vi "Main.vi"() -> ()   [LabVIEW 2013]
uses:
  <vilib>/Utility/error.llb/DialogType.ctl
panel:
  out "setPoint V 3":string
  out "setPoint I 3":string
  out "K3 conn":bool caption="NC"
  out "setPoint V 2":string
  out "setPoint I 2":string
  out "setPoint V 1":string
  out "setPoint I 1":string
  out "message 3":string=" INSTRUCTIONS:\r\rNormal Use:  When using subVIs that incorporate the error in/error out (or error I/O) structure, place this handler where you want to inform the user of an error, typically at the end of the I/O data path, as the last action of the program.  If the error in error? is ERROR, the handler creates a message describing the error and its source.  If the type of dialog = 1 (default), the message is displayed to the user, who can only acknowedge it.  If the type = 2, the user can acknowledge the message or abort execution; aborting a program with active I/O is not recommended.  If the type = 0, no message is displayed; this is used to process the error programmatically, and the error out cluster elements are wired to individual terminals for that reason.  \r\rOther Use:\n\r\nlocal testing.  To test the error code of a subVI or function that does not have the error I/O structure, you can wire its error code and a source string to the local error code and error source inputs.  If error in error? indicates no error and error code is not equal to 0, the local code and source are substituted for the error in values, and error? is set TRUE (ERROR)."
  out "conn src 3":refnum<k5>
  in  "IP 3":string="10.93.114.54"
  in  "А 3":dbl min=0.0 max=10.0 step=0.001 format="%.3f"
  in  "V 3":dbl min=0.0 max=160.0 step=0.1 format="%.1f"
  in  "NeedToSetVoltage 3":bool
  out "V 3":string
  out "А 3":string
  out "Out 2":bool
  in  "NeedToSetCurrent 3":bool
  in  "Вкл3":bool
  in  "Выкл3":bool
  in  "Выкл2":bool
  in  "Выкл":bool
  out "K2 conn":bool caption="NC"
  out "K1 conn":bool caption="NC"
  in  "IP 2":string="10.93.114.53"
  in  "IP 1":string="10.93.114.52"
  in  "А 2":dbl min=0.0 max=10.0 step=0.001 format="%.3f"
  in  "NeedToSetCurrent 2":bool
  out "V 2":string
  out "А 2":string
  in  "Вкл2":bool
  out "Out":bool
  in  "V 2":dbl min=0.0 max=160.0 step=0.1 format="%.1f"
  in  "NeedToSetVoltage 2":bool
  out "message 2":string=" INSTRUCTIONS:\r\rNormal Use:  When using subVIs that incorporate the error in/error out (or error I/O) structure, place this handler where you want to inform the user of an error, typically at the end of the I/O data path, as the last action of the program.  If the error in error? is ERROR, the handler creates a message describing the error and its source.  If the type of dialog = 1 (default), the message is displayed to the user, who can only acknowedge it.  If the type = 2, the user can acknowledge the message or abort execution; aborting a program with active I/O is not recommended.  If the type = 0, no message is displayed; this is used to process the error programmatically, and the error out cluster elements are wired to individual terminals for that reason.  \r\rOther Use:\n\r\nlocal testing.  To test the error code of a subVI or function that does not have the error I/O structure, you can wire its error code and a source string to the local error code and error source inputs.  If error in error? indicates no error and error code is not equal to 0, the local code and source are substituted for the error in values, and error? is set TRUE (ERROR)."
  out "conn src 2":refnum<k5>
  out "conn src":refnum<k5>
  in  "stop":bool
  out "message":string=" INSTRUCTIONS:\r\rNormal Use:  When using subVIs that incorporate the error in/error out (or error I/O) structure, place this handler where you want to inform the user of an error, typically at the end of the I/O data path, as the last action of the program.  If the error in error? is ERROR, the handler creates a message describing the error and its source.  If the type of dialog = 1 (default), the message is displayed to the user, who can only acknowedge it.  If the type = 2, the user can acknowledge the message or abort execution; aborting a program with active I/O is not recommended.  If the type = 0, no message is displayed; this is used to process the error programmatically, and the error out cluster elements are wired to individual terminals for that reason.  \r\rOther Use:\n\r\nlocal testing.  To test the error code of a subVI or function that does not have the error I/O structure, you can wire its error code and a source string to the local error code and error source inputs.  If error in error? indicates no error and error code is not equal to 0, the local code and source are substituted for the error in values, and error? is set TRUE (ERROR)."
  in  "V":dbl min=0.0 max=160.0 step=0.1 format="%.1f"
  in  "А":dbl min=0.0 max=10.0 step=0.001 format="%.3f"
  in  "NeedToSetVoltage":bool
  in  "NeedToSetCurrent":bool
  out "V":string
  out "А":string
  in  "Вкл.":bool
  out "Out":bool
  # "1"
  # "Settings"
  # "Setpoint"
  # "2"
  # "Settings"
  # "Setpoint"
  # "3"
  # "Settings"
  # "Setpoint"
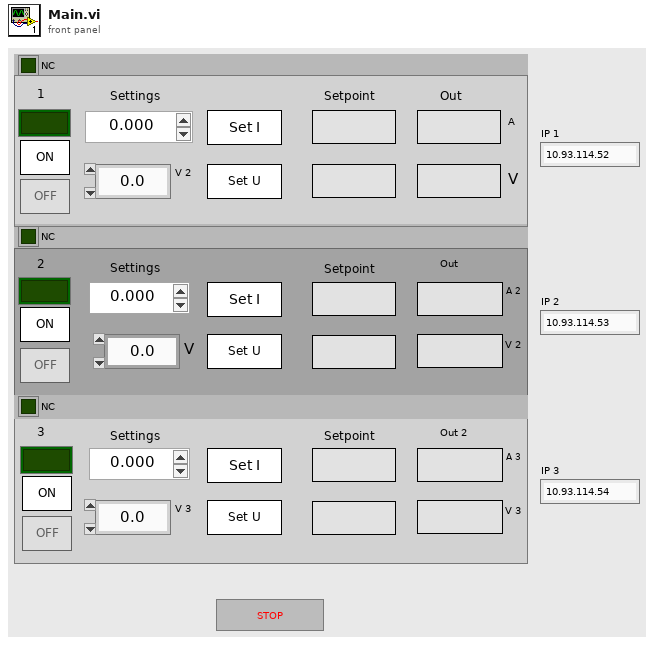
[diagram p1: front panel]
types:
  T1 = enum8{"Enabled", "Disabled", "Disabled and Grayed Out"}
  T2 = typedef "DialogType.ctl" = u16
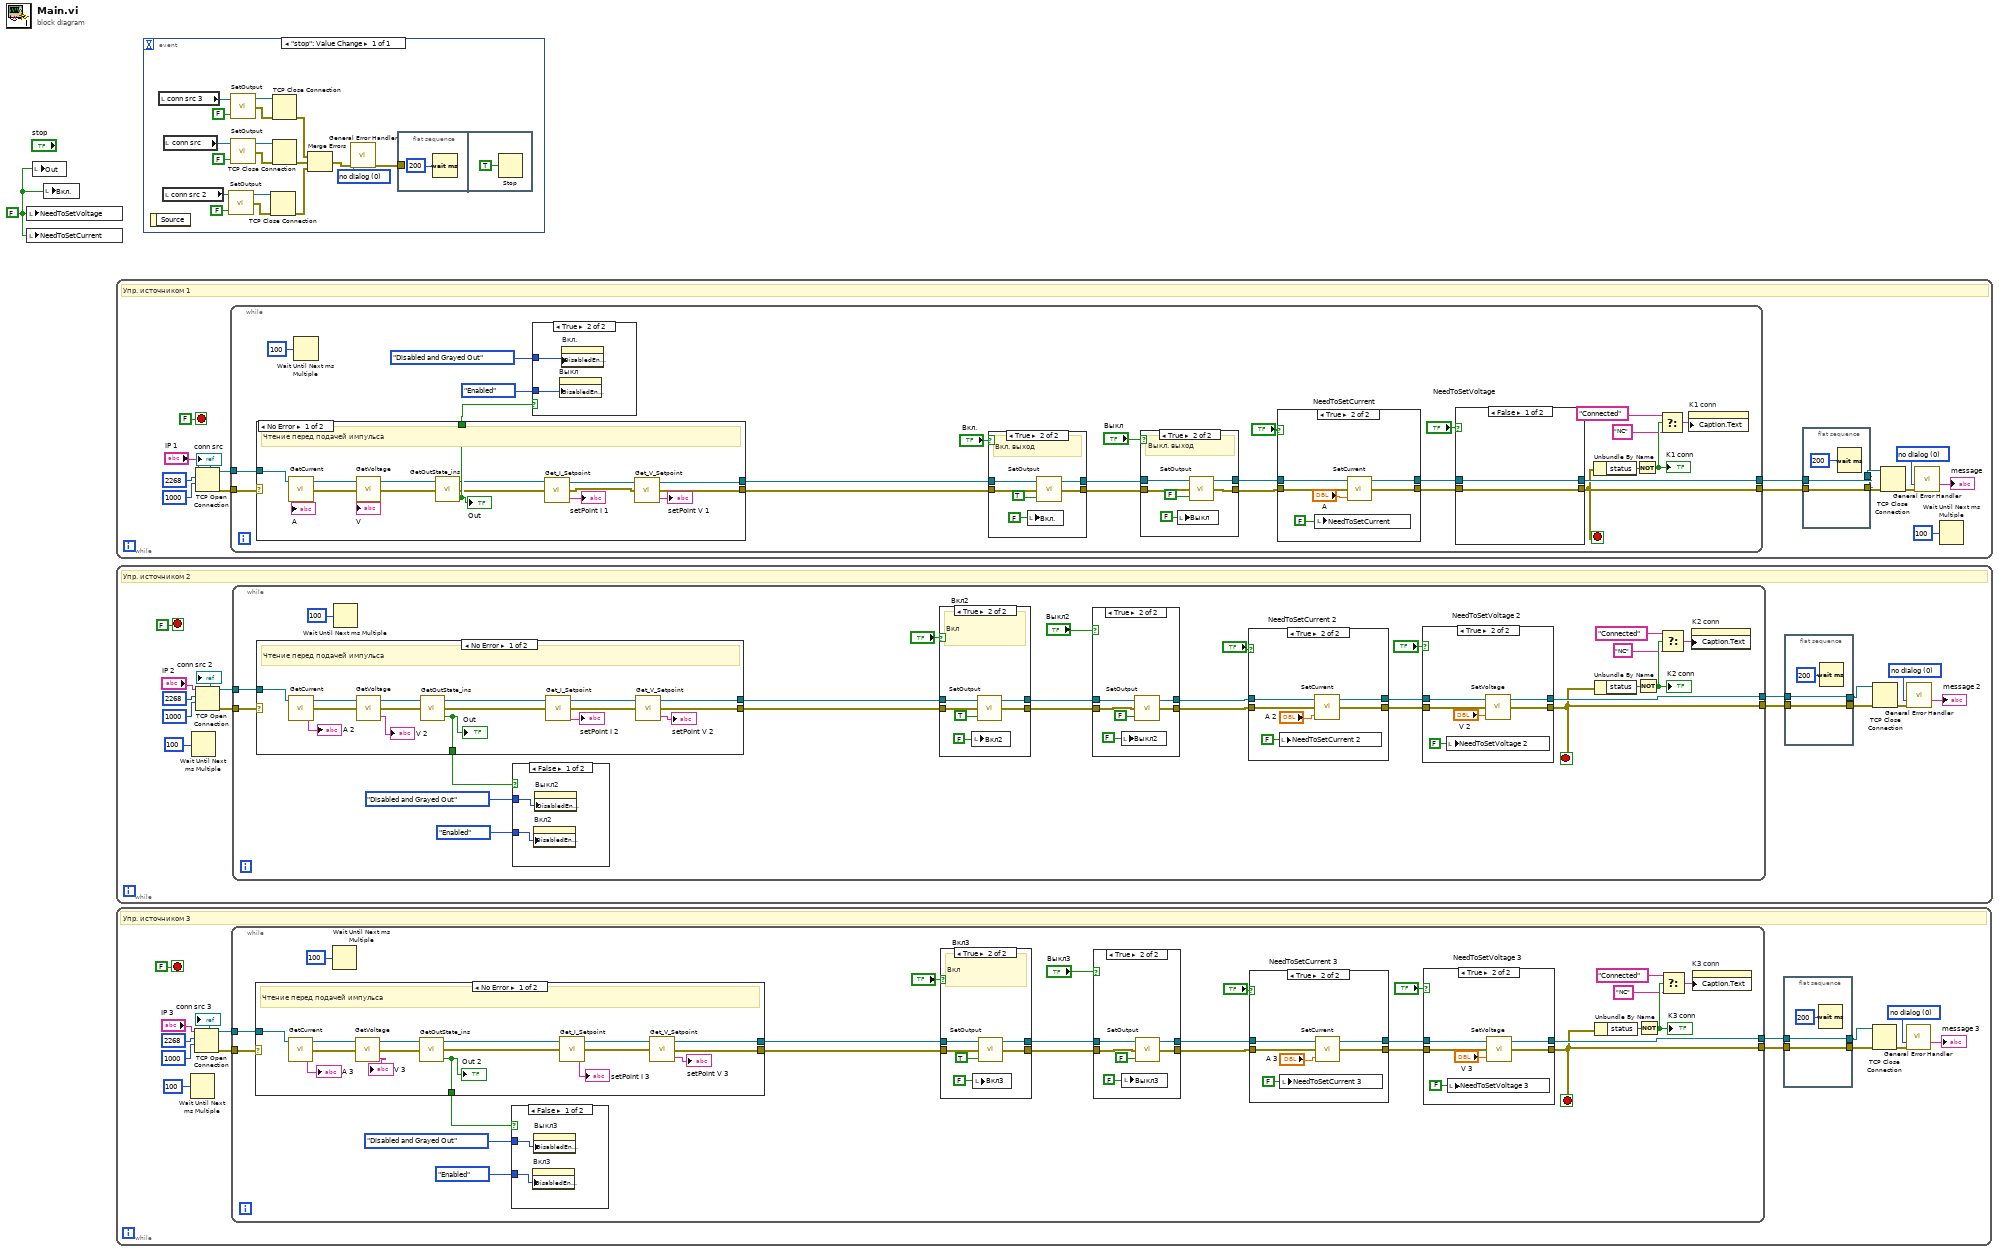
[diagram p0: block diagram]
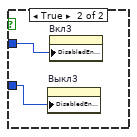
[diagram p3: hidden frame]
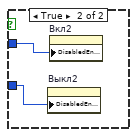
[diagram p9: hidden frame]
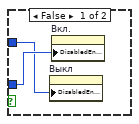
[diagram p15: hidden frame]
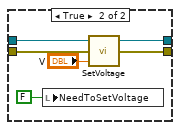
[diagram p19: hidden frame]
diagram:
  w1 = FALSE ("Connect")
  n1 = local write "NeedToSetVoltage"(w1) -> ()
  n2 = local write "NeedToSetCurrent"(w1) -> ()
  n3 = local write "Out"(w1) -> ()
  n4 = local write "Вкл."(w1) -> ()
  n5 = while {
    stop <- FALSE stop-if-true
    w10 = T2 0 items=["no dialog", "OK message", "continue or stop message", "OK message + warnings", "continue/stop + warnings"] ("type of dialog (OK msg:1)")
    # "Упр. источником 3"
    n6 = Wait Until Next ms Multiple(millisecond multiple=u32 100 ("milliseconds to wait")) -> ()  [unwired: 1 out]
    n7 = TCP Open Connection(address="IP 3", remote port or service name=u16 2268 ("Port"), timeout ms (60000)=1000) -> (connection ID=w12:refnum<k5>, error out=w13:errorcluster)  [unwired: 1 in, 1 out]
    "conn src 3" <- w12
    n8 = while {
      tunnel: w13 -> [w43]
      tunnel: w12 -> [w42]
      tunnel: [w41] -> w5
      tunnel: [w27] -> w3
      stop <- w27 stop-if-true
      n9 = case shown="No Error" w43 {
        selector: w43 -> [_ w80]
        tunnel: w42 -> [w77 w81]
        tunnel: [w68 w80] -> w37
        tunnel: [w69 w81] -> w36
        tunnel: [w72 _] -> w24
        frame No Error {
          # "Чтение перед подачей импульса"
          n10 = call "GetCurrent.vi"("connection ID"=w77) -> ("Current"=→"А 3":string, "error out"=w78:errorcluster, "connection ID out"=w79:refnum<k5>)  [unwired: 1 in, 1 out]
          n11 = call "GetVoltage.vi"("error in"=w78, "connection ID"=w79) -> ("Voltage"=→"V 3":string, "error out"=w73:errorcluster, "connection ID out"=w74:refnum<k5>)  [unwired: 1 out]
          n12 = call "GetOutState_ins.vi"("error in"=w73, "connection ID"=w74) -> ("OutState"=w72:bool, "error out"=w66:errorcluster, "connection ID out"=w71:refnum<k5>)  [unwired: 1 out]
          "Out 2" <- w72
          n13 = call "Get_I_Setpoint.vi"("error in"=w66, "connection ID"=w71) -> ("I setpoint"=→"setPoint I 3":string, "error out"=w67:errorcluster, "connection ID out"=w70:refnum<k5>)  [unwired: 1 out]
          n14 = call "Get_V_Setpoint.vi"("error in"=w67, "connection ID"=w70) -> ("v setpoint"=→"setPoint V 3":string, "error out"=w68:errorcluster, "connection ID out"=w69:refnum<k5>)  [unwired: 1 out]
        }
        frame Error {
        }
      }
      n15 = Wait Until Next ms Multiple(millisecond multiple=u32 100) -> ()  [unwired: 1 out]
      n16 = case shown="False" w24 {
        tunnel: T1."Disabled and Grayed Out" ("Disabled") -> [w52 w55]
        tunnel: T1."Enabled" ("Disabled") -> [w53 w54]
        frame False {
          n17 = property on="Вкл3" class="Bool (strict)"("DisabledEnum"=w53) -> ()  [unwired: 2 in, 2 out]
          n18 = property on="Выкл3" class="Bool (strict)"("DisabledEnum"=w52) -> ()  [unwired: 2 in, 2 out]
        }
        frame True {
          n19 = property on="Выкл3" class="Bool (strict)"("DisabledEnum"=w54) -> ()  [unwired: 2 in, 2 out]
          n20 = property on="Вкл3" class="Bool (strict)"("DisabledEnum"=w55) -> ()  [unwired: 2 in, 2 out]
        }
      }
      n21 = case shown="True" "Вкл3" {
        tunnel: w37 -> [w56 w63]
        tunnel: w36 -> [w57 w62]
        tunnel: [w57 w61] -> w22
        tunnel: [w56 w60] -> w21
        frame False {
          # "Вкл."
        }
        frame True {
          # "Вкл"
          n22 = local write "Вкл3"(FALSE ("Вкл2")) -> ()
          n23 = call "SetOutput.vi"("State"=TRUE, "error in"=w63, "connection ID"=w62) -> ("error out"=w60:errorcluster, "connection ID out"=w61:refnum<k5>)  [unwired: 1 out]
        }
      }
      n24 = case shown="True" "Выкл3" {
        tunnel: w22 -> [w45 w50]
        tunnel: w21 -> [w44 w49]
        tunnel: [w45 w48] -> w20
        tunnel: [w44 w47] -> w19
        frame False {
        }
        frame True {
          n25 = local write "Выкл3"(FALSE ("Выкл2")) -> ()
          n26 = call "SetOutput.vi"("State"=FALSE, "error in"=w49, "connection ID"=w50) -> ("error out"=w47:errorcluster, "connection ID out"=w48:refnum<k5>)  [unwired: 1 out]
        }
      }
      n27 = case shown="True" "NeedToSetCurrent 3" {
        tunnel: [w91 w97] -> w40
        tunnel: [w90 w95] -> w38
        tunnel: w20 -> [w91 w94]
        tunnel: w19 -> [w90 w93]
        frame False {
        }
        frame True {
          n28 = local write "NeedToSetCurrent 3"(FALSE ("NeedToSetOutput")) -> ()
          n29 = call "SetCurrent.vi"("Current"="А 3", "error in"=w93, "connection ID"=w94) -> ("error out"=w95:errorcluster, "connection ID out"=w97:refnum<k5>)  [unwired: 1 out]
        }
      }
      n30 = case shown="True" "NeedToSetVoltage 3" {
        tunnel: w40 -> [w83 w89]
        tunnel: [w83 w86] -> w41
        tunnel: w38 -> [w82 w85]
        tunnel: [w82 w84] -> w27
        frame False {
        }
        frame True {
          n31 = local write "NeedToSetVoltage 3"(FALSE ("NeedToSetOutput")) -> ()
          n32 = call "SetVoltage.vi"("Voltage"="V 3", "error in"=w85, "connection ID"=w89) -> ("error out"=w84:errorcluster, "connection ID out"=w86:refnum<k5>)  [unwired: 1 out]
        }
      }
      n33 = Unbundle By Name(w27) -> ("status"=w32:bool)
      n34 = Not(x=w32) -> (.not. x?=w31:bool)
      "K3 conn" <- w31
      n35 = Select(t="Connected", s=w31, f="NC") -> (s? t:f=w30:string)
      n36 = property on="K3 conn" class="Bool (strict)"("Caption.Text"=w30) -> ()  [unwired: 2 in, 2 out]
    }
    n37 = flat-sequence {
      tunnel: [w18] -> w4
      tunnel: w5 -> [w18]
      tunnel: w3 -> [w17]
      tunnel: [w17] -> w2
      frame #0 {
        n38 = Wait (ms)(milliseconds to wait=u32 200 ("millisecond multiple")) -> ()  [unwired: 1 out]
      }
    }
    n39 = TCP Close Connection(connection ID=w4, error in (no error)=w2) -> (error out=w11:errorcluster)  [unwired: 2 out]
    n40 = call <vilib>:"General Error Handler.vi"("type of dialog (OK msg:1)"=w10, "error in (no error)"=w11) -> ("message"=→"message 3":string)  [unwired: 9 in, 4 out]
  }
  n41 = while {
    stop <- FALSE stop-if-true
    w106 = T2 0 items=["no dialog", "OK message", "continue or stop message", "OK message + warnings", "continue/stop + warnings"] ("type of dialog (OK msg:1)")
    # "Упр. источником 1"
    n42 = TCP Open Connection(address="IP 1", remote port or service name=u16 2268 ("Port"), timeout ms (60000)=1000) -> (connection ID=w108:refnum<k5>, error out=w109:errorcluster)  [unwired: 1 in, 1 out]
    "conn src" <- w108
    n43 = while {
      tunnel: w109 -> [w139]
      tunnel: w108 -> [w138]
      tunnel: [w137] -> w101
      tunnel: [w128] -> w100
      stop <- w128 stop-if-true
      n44 = case shown="No Error" w139 {
        selector: w139 -> [_ w184]
        tunnel: w138 -> [w179 w185]
        tunnel: [w170 w184] -> w133
        tunnel: [w171 w185] -> w132
        tunnel: [w176 _] -> w122
        frame No Error {
          # "Чтение перед подачей импульса"
          n45 = call "GetCurrent.vi"("connection ID"=w179) -> ("Current"=→"А":string, "error out"=w180:errorcluster, "connection ID out"=w182:refnum<k5>)  [unwired: 1 in, 1 out]
          n46 = call "GetVoltage.vi"("error in"=w180, "connection ID"=w182) -> ("Voltage"=→"V":string, "error out"=w178:errorcluster, "connection ID out"=w177:refnum<k5>)  [unwired: 1 out]
          n47 = call "GetOutState_ins.vi"("error in"=w178, "connection ID"=w177) -> ("OutState"=w176:bool, "error out"=w175:errorcluster, "connection ID out"=w174:refnum<k5>)  [unwired: 1 out]
          "Out" <- w176
          n48 = call "Get_I_Setpoint.vi"("error in"=w175, "connection ID"=w174) -> ("I setpoint"=→"setPoint I 1":string, "error out"=w168:errorcluster, "connection ID out"=w172:refnum<k5>)  [unwired: 1 out]
          n49 = call "Get_V_Setpoint.vi"("error in"=w168, "connection ID"=w172) -> ("v setpoint"=→"setPoint V 1":string, "error out"=w170:errorcluster, "connection ID out"=w171:refnum<k5>)  [unwired: 1 out]
        }
        frame Error {
        }
      }
      n50 = Wait Until Next ms Multiple(millisecond multiple=u32 100) -> ()  [unwired: 1 out]
      n51 = case shown="True" w122 {
        tunnel: T1."Enabled" ("Disabled") -> [w149 w151]
        tunnel: T1."Disabled and Grayed Out" ("Disabled") -> [w148 w150]
        frame False {
          n52 = property on="Выкл" class="Bool (strict)"("DisabledEnum"=w148) -> ()  [unwired: 2 in, 2 out]
          n53 = property on="Вкл." class="Bool (strict)"("DisabledEnum"=w149) -> ()  [unwired: 2 in, 2 out]
        }
        frame True {
          n54 = property on="Выкл" class="Bool (strict)"("DisabledEnum"=w151) -> ()  [unwired: 2 in, 2 out]
          n55 = property on="Вкл." class="Bool (strict)"("DisabledEnum"=w150) -> ()  [unwired: 2 in, 2 out]
        }
      }
      n56 = case shown="True" "Вкл." {
        tunnel: w133 -> [w160 w167]
        tunnel: w132 -> [w161 w166]
        tunnel: [w161 w165] -> w118
        tunnel: [w160 w164] -> w117
        frame False {
          # "Ручное управление выходом"
        }
        frame True {
          # "Вкл. выход"
          n57 = local write "Вкл."(FALSE ("Вкл.")) -> ()
          n58 = call "SetOutput.vi"("State"=TRUE, "error in"=w167, "connection ID"=w166) -> ("error out"=w164:errorcluster, "connection ID out"=w165:refnum<k5>)  [unwired: 1 out]
        }
      }
      n59 = case shown="True" "Выкл" {
        tunnel: w117 -> [w140 w147]
        tunnel: w118 -> [w141 w146]
        tunnel: [w141 w145] -> w116
        tunnel: [w140 w144] -> w115
        frame False {
          # "Ручное управление выходом"
        }
        frame True {
          # "Выкл. выход"
          n60 = local write "Выкл"(FALSE ("Вкл.")) -> ()
          n61 = call "SetOutput.vi"("State"=FALSE, "error in"=w147, "connection ID"=w146) -> ("error out"=w144:errorcluster, "connection ID out"=w145:refnum<k5>)  [unwired: 1 out]
        }
      }
      n62 = case shown="True" "NeedToSetCurrent" {
        tunnel: [w153 w158] -> w136
        tunnel: [w152 w156] -> w134
        tunnel: w116 -> [w153 w155]
        tunnel: w115 -> [w152 w154]
        frame False {
        }
        frame True {
          n63 = local write "NeedToSetCurrent"(FALSE ("NeedToSetOutput")) -> ()
          n64 = call "SetCurrent.vi"("Current"="А", "error in"=w154, "connection ID"=w155) -> ("error out"=w156:errorcluster, "connection ID out"=w158:refnum<k5>)  [unwired: 1 out]
        }
      }
      n65 = case shown="False" "NeedToSetVoltage" {
        tunnel: w136 -> [w187 w193]
        tunnel: [w187 w190] -> w137
        tunnel: w134 -> [w186 w189]
        tunnel: [w186 w188] -> w128
        frame False {
        }
        frame True {
          n66 = local write "NeedToSetVoltage"(FALSE ("NeedToSetOutput")) -> ()
          n67 = call "SetVoltage.vi"("Voltage"="V", "error in"=w189, "connection ID"=w193) -> ("error out"=w188:errorcluster, "connection ID out"=w190:refnum<k5>)  [unwired: 1 out]
        }
      }
      n68 = Unbundle By Name(w128) -> ("status"=w127:bool)
      n69 = Not(x=w127) -> (.not. x?=w126:bool)
      "K1 conn" <- w126
      n70 = Select(t="Connected", s=w126, f="NC") -> (s? t:f=w125:string)
      n71 = property on="K1 conn" class="Bool (strict)"("Caption.Text"=w125) -> ()  [unwired: 2 in, 2 out]
    }
    n72 = flat-sequence {
      tunnel: [w114] -> w102
      tunnel: w101 -> [w114]
      tunnel: [w113] -> w99
      tunnel: w100 -> [w113]
      frame #0 {
        n73 = Wait (ms)(milliseconds to wait=u32 200 ("millisecond multiple")) -> ()  [unwired: 1 out]
      }
    }
    n74 = TCP Close Connection(connection ID=w102, error in (no error)=w99) -> (error out=w107:errorcluster)  [unwired: 2 out]
    n75 = call <vilib>:"General Error Handler.vi"("type of dialog (OK msg:1)"=w106, "error in (no error)"=w107) -> ("message"=→"message":string)  [unwired: 9 in, 4 out]
    n76 = Wait Until Next ms Multiple(millisecond multiple=u32 100) -> ()  [unwired: 1 out]
  }
  n77 = while {
    stop <- FALSE stop-if-true
    w202 = T2 0 items=["no dialog", "OK message", "continue or stop message", "OK message + warnings", "continue/stop + warnings"] ("type of dialog (OK msg:1)")
    # "Упр. источником 2"
    n78 = Wait Until Next ms Multiple(millisecond multiple=u32 100 ("milliseconds to wait")) -> ()  [unwired: 1 out]
    n79 = TCP Open Connection(address="IP 2", remote port or service name=u16 2268 ("Port"), timeout ms (60000)=1000) -> (connection ID=w204:refnum<k5>, error out=w205:errorcluster)  [unwired: 1 in, 1 out]
    "conn src 2" <- w204
    n80 = while {
      tunnel: w205 -> [w235]
      tunnel: w204 -> [w234]
      tunnel: [w233] -> w197
      tunnel: [w219] -> w195
      stop <- w219 stop-if-true
      n81 = case shown="No Error" w235 {
        selector: w235 -> [_ w272]
        tunnel: w234 -> [w269 w273]
        tunnel: [w258 w272] -> w229
        tunnel: [w259 w273] -> w228
        tunnel: [w265 _] -> w216
        frame No Error {
          # "Чтение перед подачей импульса"
          n82 = call "GetCurrent.vi"("connection ID"=w269) -> ("Current"=→"А 2":string, "error out"=w270:errorcluster, "connection ID out"=w271:refnum<k5>)  [unwired: 1 in, 1 out]
          n83 = call "GetVoltage.vi"("error in"=w270, "connection ID"=w271) -> ("Voltage"=→"V 2":string, "error out"=w266:errorcluster, "connection ID out"=w267:refnum<k5>)  [unwired: 1 out]
          n84 = call "GetOutState_ins.vi"("error in"=w266, "connection ID"=w267) -> ("OutState"=w265:bool, "error out"=w262:errorcluster, "connection ID out"=w263:refnum<k5>)  [unwired: 1 out]
          "Out" <- w265
          n85 = call "Get_I_Setpoint.vi"("error in"=w262, "connection ID"=w263) -> ("I setpoint"=→"setPoint I 2":string, "error out"=w261:errorcluster, "connection ID out"=w260:refnum<k5>)  [unwired: 1 out]
          n86 = call "Get_V_Setpoint.vi"("error in"=w261, "connection ID"=w260) -> ("v setpoint"=→"setPoint V 2":string, "error out"=w258:errorcluster, "connection ID out"=w259:refnum<k5>)  [unwired: 1 out]
        }
        frame Error {
        }
      }
      n87 = Wait Until Next ms Multiple(millisecond multiple=u32 100) -> ()  [unwired: 1 out]
      n88 = case shown="False" w216 {
        tunnel: T1."Disabled and Grayed Out" ("Disabled") -> [w244 w247]
        tunnel: T1."Enabled" ("Disabled") -> [w245 w246]
        frame False {
          n89 = property on="Вкл2" class="Bool (strict)"("DisabledEnum"=w245) -> ()  [unwired: 2 in, 2 out]
          n90 = property on="Выкл2" class="Bool (strict)"("DisabledEnum"=w244) -> ()  [unwired: 2 in, 2 out]
        }
        frame True {
          n91 = property on="Выкл2" class="Bool (strict)"("DisabledEnum"=w246) -> ()  [unwired: 2 in, 2 out]
          n92 = property on="Вкл2" class="Bool (strict)"("DisabledEnum"=w247) -> ()  [unwired: 2 in, 2 out]
        }
      }
      n93 = case shown="True" "Вкл2" {
        tunnel: w229 -> [w248 w255]
        tunnel: w228 -> [w249 w254]
        tunnel: [w249 w253] -> w214
        tunnel: [w248 w252] -> w213
        frame False {
          # "Вкл."
        }
        frame True {
          # "Вкл"
          n94 = local write "Вкл2"(FALSE ("Вкл2")) -> ()
          n95 = call "SetOutput.vi"("State"=TRUE, "error in"=w255, "connection ID"=w254) -> ("error out"=w252:errorcluster, "connection ID out"=w253:refnum<k5>)  [unwired: 1 out]
        }
      }
      n96 = case shown="True" "Выкл2" {
        tunnel: w214 -> [w237 w242]
        tunnel: w213 -> [w236 w241]
        tunnel: [w237 w240] -> w212
        tunnel: [w236 w239] -> w211
        frame False {
        }
        frame True {
          n97 = local write "Выкл2"(FALSE ("Выкл2")) -> ()
          n98 = call "SetOutput.vi"("State"=FALSE, "error in"=w241, "connection ID"=w242) -> ("error out"=w239:errorcluster, "connection ID out"=w240:refnum<k5>)  [unwired: 1 out]
        }
      }
      n99 = case shown="True" "NeedToSetCurrent 2" {
        tunnel: [w283 w289] -> w232
        tunnel: [w282 w287] -> w230
        tunnel: w212 -> [w283 w286]
        tunnel: w211 -> [w282 w285]
        frame False {
        }
        frame True {
          n100 = local write "NeedToSetCurrent 2"(FALSE ("NeedToSetOutput")) -> ()
          n101 = call "SetCurrent.vi"("Current"="А 2", "error in"=w285, "connection ID"=w286) -> ("error out"=w287:errorcluster, "connection ID out"=w289:refnum<k5>)  [unwired: 1 out]
        }
      }
      n102 = case shown="True" "NeedToSetVoltage 2" {
        tunnel: w232 -> [w275 w281]
        tunnel: [w275 w278] -> w233
        tunnel: w230 -> [w274 w277]
        tunnel: [w274 w276] -> w219
        frame False {
        }
        frame True {
          n103 = local write "NeedToSetVoltage 2"(FALSE ("NeedToSetOutput")) -> ()
          n104 = call "SetVoltage.vi"("Voltage"="V 2", "error in"=w277, "connection ID"=w281) -> ("error out"=w276:errorcluster, "connection ID out"=w278:refnum<k5>)  [unwired: 1 out]
        }
      }
      n105 = Unbundle By Name(w219) -> ("status"=w224:bool)
      n106 = Not(x=w224) -> (.not. x?=w223:bool)
      "K2 conn" <- w223
      n107 = Select(t="Connected", s=w223, f="NC") -> (s? t:f=w222:string)
      n108 = property on="K2 conn" class="Bool (strict)"("Caption.Text"=w222) -> ()  [unwired: 2 in, 2 out]
    }
    n109 = flat-sequence {
      tunnel: [w210] -> w196
      tunnel: w197 -> [w210]
      tunnel: w195 -> [w209]
      tunnel: [w209] -> w194
      frame #0 {
        n110 = Wait (ms)(milliseconds to wait=u32 200 ("millisecond multiple")) -> ()  [unwired: 1 out]
      }
    }
    n111 = TCP Close Connection(connection ID=w196, error in (no error)=w194) -> (error out=w203:errorcluster)  [unwired: 2 out]
    n112 = call <vilib>:"General Error Handler.vi"("type of dialog (OK msg:1)"=w202, "error in (no error)"=w203) -> ("message"=→"message 2":string)  [unwired: 9 in, 4 out]
  }
  n113 = event shown="[0] \"stop\": Value Change" {
    selector: _ -> [_]
    dyn-events: _ -> [_]
    timeout: _ -> [_]
    event "stop": Value Change {
      w305 = T2 0 items=["no dialog", "OK message", "continue or stop message", "OK message + warnings", "continue/stop + warnings"] ("type of dialog (OK msg:1)")
      n114 = event-data() -> ()  [unwired: 1 in, 1 out]
      n115 = local read "conn src 3"() -> (w291:refnum<k5>)
      n116 = local read "conn src 2"() -> (w296:refnum<k5>)
      n117 = local read "conn src"() -> (w303:refnum<k5>)
      n118 = call "SetOutput.vi"("State"=FALSE, "connection ID"=w296) -> ("error out"=w298:errorcluster, "connection ID out"=w297:refnum<k5>)  [unwired: 1 in, 1 out]
      n119 = call "SetOutput.vi"("State"=FALSE, "connection ID"=w291) -> ("error out"=w293:errorcluster, "connection ID out"=w292:refnum<k5>)  [unwired: 1 in, 1 out]
      n120 = call "SetOutput.vi"("State"=FALSE, "connection ID"=w303) -> ("error out"=w301:errorcluster, "connection ID out"=w302:refnum<k5>)  [unwired: 1 in, 1 out]
      n121 = TCP Close Connection(connection ID=w297, error in (no error)=w298) -> (error out=w295:errorcluster)  [unwired: 1 in, 1 out]
      n122 = TCP Close Connection(connection ID=w292, error in (no error)=w293) -> (error out=w290:errorcluster)  [unwired: 1 in, 1 out]
      n123 = TCP Close Connection(connection ID=w302, error in (no error)=w301) -> (error out=w307:errorcluster)  [unwired: 1 in, 1 out]
      n124 = Merge Errors(w290, w307, w295) -> (w306:errorcluster)
      n125 = call <vilib>:"General Error Handler.vi"("type of dialog (OK msg:1)"=w305, "error in (no error)"=w306) -> ("error out"=w304:errorcluster)  [unwired: 9 in, 4 out]
      n126 = flat-sequence {
        tunnel: w304 -> [_]
        frame #0 {
          n127 = Wait (ms)(milliseconds to wait=u32 200) -> ()  [unwired: 1 out]
        }
        frame #1 {
          n128 = Stop(stop? (T)=TRUE) -> ()
        }
      }
    }
  }
